vi "GetNotifierRef.vi"(8 "error in (no error)":errorcluster, 11 "WindowFrame in":refnum<class "WindowFrame.lvclass">) -> (0 "error out":errorcluster, 2 "NotifierRef":refnum<notifier>, 3 "WindowFrame out":refnum<class "WindowFrame.lvclass">)   [LabVIEW 2021]
uses:
  WindowFrame.lvclass/WindowFrame.ctl
  351abfd1-6ef3-46a3-81e9-bcf8ed5a4216.vi
  WindowFrame.lvclass
  C:/Users/Dany/OneDrive/LabVIEW/Class/ClassUtilities/ClassByRef/ClassByRef.lvclass
  C:/Users/Dany/OneDrive/LabVIEW/Class/WindowFrame/WindowFrame.lvclass
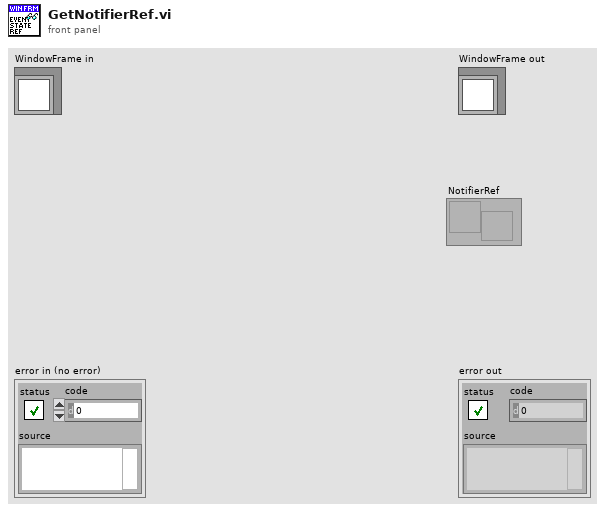
[diagram p1: front panel]
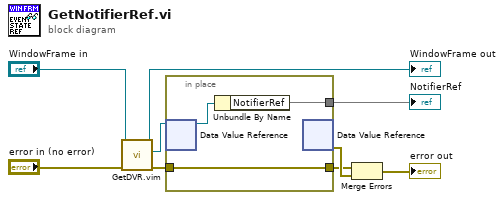
[diagram p0: block diagram]
diagram:
  n1 = call "GetDVR.vim"("error in (no error)"="error in (no error)", "ByRefClass in"="WindowFrame in") -> ("error out"=w2:errorcluster, "DVR"=w1:refnum<data-value>, "ByRefClass out"=→"WindowFrame out":refnum<class "WindowFrame.lvclass">)  [unwired: 7 in]
  n2 = in-place {
    in-place-border: w2 -> [w12]
    in-place-border: [w12] -> w3
    in-place-border: [w10] -> w5
    n3 = in-place-dvr #1(w1) -> (w11:refnum<class "WindowFrame.lvclass">)  [unwired: 1 out]
    n4 = Unbundle By Name(w11) -> ("NotifierRef"=w10)
    n5 = in-place-dvr #1() -> (w4:errorcluster)  [unwired: 1 in, 1 out]
  }
  "NotifierRef" <- w5
  n6 = Merge Errors(w3, w4) -> (→"error out":errorcluster)
